vi "horizontal mag adjust.vi"(8 "y":bool=TRUE, 9 "x":bool=TRUE, 10 "2D mag correct":dbl, 11 "Array in":u16[][](array[numeric])) -> (3 "Array out":u16[][](array[numeric]))   [LabVIEW 2024]
uses:
  <vilib>/vision/NI_Vision_Development_Module.lvlib
panel:
  in  "Interpolation Type":u32(ring)=1 items=["Zero Order", "Bi-Linear", "Quadratic", "Cubic Spline"]
  out "x-y":dbl
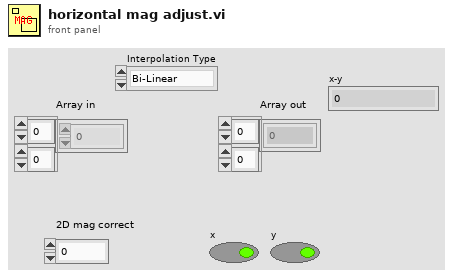
[diagram p1: front panel]
types:
  T1 = typedef "Image Type" = u32
  T2 = typedef "IMAQ Image.ctl" = refnum<image>
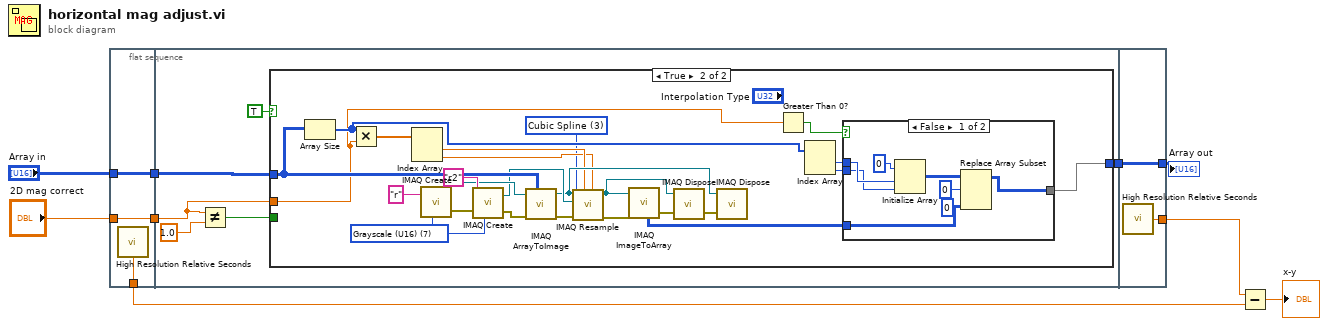
[diagram p0: block diagram]
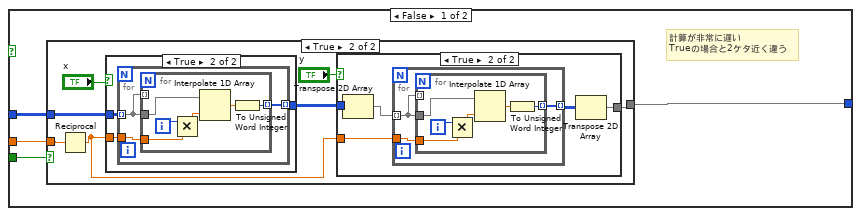
[diagram p2: hidden frame]
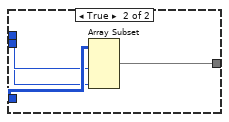
[diagram p6: hidden frame]
diagram:
  n1 = flat-sequence {
    tunnel: "2D mag correct" -> [w11]
    tunnel: "Array in" -> [w12]
    tunnel: [w12] -> w7
    tunnel: [w11] -> w6
    tunnel: [w10] -> w4
    tunnel: [w16] -> w8
    tunnel: w7 -> [w15]
    tunnel: w6 -> [w14]
    tunnel: [w97] -> w2
    tunnel: w8 -> [w97]
    tunnel: [w96] -> w5
    frame #0 {
      n2 = call <vilib>:"High Resolution Relative Seconds.vi"() -> ("relative seconds"=w10:dbl)
    }
    frame #1 {
      n3 = Not Equal?(x=w14, y=1.0) -> (x != y?=w18:bool)
      n4 = case shown="True" TRUE {
        tunnel: w18 -> [w22 _]
        tunnel: [w21 w65] -> w16
        tunnel: w15 -> [w20 w80]
        tunnel: w14 -> [w19 w60]
        frame False {
          # "計算が非常に遅い\nTrueの場合と2ケタ近く違う"
          n5 = case shown="True" w22 {
            tunnel: w20 -> [w23 w30]
            tunnel: [w23 w28] -> w21
            tunnel: w19 -> [_ w25]
            frame False {
            }
            frame True {
              n6 = Reciprocal(x=w25) -> (1/x=w24:dbl)
              n7 = case shown="True" "x" {
                tunnel: w30 -> [w31 w34]
                tunnel: [w31 w33] -> w29
                tunnel: w24 -> [_ w32]
                frame False {
                }
                frame True {
                  n8 = for {
                    tunnel: w34 -> [w36] mode=indexing
                    tunnel: w32 -> [w37]
                    tunnel: [w35] -> w33 mode=indexing
                    n9 = for {
                      tunnel: w36 -> [w41]
                      tunnel: w37 -> [w42]
                      tunnel: [w38] -> w35 mode=indexing
                      tunnel: w36 -> [_] mode=indexing
                      i -> [w43]
                      n10 = Multiply(x=w43, y=w42) -> (x*y=w40:dbl)
                      n11 = Interpolate 1D Array(1:w40, 2:w41) -> (0:w39:dbl)
                      n12 = To Unsigned Word Integer(number=w39) -> (unsigned 16bit integer=w38:u16)
                    }
                  }
                }
              }
              n13 = case shown="True" "y" {
                tunnel: w29 -> [w44 w49]
                tunnel: [w44 w46] -> w28
                tunnel: w24 -> [_ w45]
                frame False {
                }
                frame True {
                  n14 = Transpose 2D Array(2D array=w49) -> (transposed array=w48:u16[][])
                  n15 = for {
                    tunnel: w48 -> [w51] mode=indexing
                    tunnel: w45 -> [w52]
                    tunnel: [w50] -> w47 mode=indexing
                    n16 = for {
                      tunnel: w51 -> [w56]
                      tunnel: w52 -> [w57]
                      tunnel: [w53] -> w50 mode=indexing
                      tunnel: w51 -> [_] mode=indexing
                      i -> [w58]
                      n17 = Multiply(x=w58, y=w57) -> (x*y=w55:dbl)
                      n18 = Interpolate 1D Array(1:w55, 2:w56) -> (0:w54:dbl)
                      n19 = To Unsigned Word Integer(number=w54) -> (unsigned 16bit integer=w53:u16)
                    }
                  }
                  n20 = Transpose 2D Array(2D array=w47) -> (transposed array=w46:u16[][])
                }
              }
            }
          }
        }
        frame True {
          w59 = u32 3 items=["Zero Order", "Bi-Linear", "Quadratic", "Cubic Spline"] ("Interpolation Type")
          w76 = T1 7 items=["Grayscale (U8)", "Grayscale (I16)", "Grayscale (SGL)", "Complex (CSG)", "RGB (U32)", "HSL (U32)", "RGB (U64)", "Grayscale (U16)"] ("Image Type")
          n21 = Array Size(array=w80) -> (size(s)=w64:i32[])
          n22 = Multiply(x=w64, y=w60) -> (x*y=w81:dbl[])
          n23 = Index Array(array=w81) -> (element #1=w67:dbl, element #2=w66:dbl)  [unwired: 2 in]
          n24 = call "IMAQ Create"("Image Name"="r", "Image Type"=w76) -> ("New Image"=w74:T2, "error out"=w77:errorcluster)  [unwired: 3 in]
          n25 = call "IMAQ Create"("Image Name"="r2", "Image Type"=w76, "error in (no error)"=w77) -> ("New Image"=w71:T2, "error out"=w75:errorcluster)  [unwired: 2 in]
          n26 = call "IMAQ ArrayToImage"("Image Pixels (U16)"=w80, "error in (no error)"=w75, "Image"=w74) -> ("error out"=w73:errorcluster, "Image Out"=w69:T2)  [unwired: 7 in]
          n27 = call "IMAQ Resample"("X Resolution"=w66, "Y Resolution"=w67, "error in (no error)"=w73, "Interpolation Type"=w59, "Image Dst"=w71, "Image Src"=w69) -> ("error out"=w72:errorcluster, "Image Dst Out"=w70:T2)  [unwired: 4 in]
          n28 = call "IMAQ ImageToArray"("error in (no error)"=w72, "Image"=w70) -> ("Image Pixels (U16)"=w68:u16[][], "error out"=w83:errorcluster)  [unwired: 2 in, 3 out]
          n29 = call "IMAQ Dispose"("Image"=w70, "error in (no error)"=w83) -> ("error out"=w79:errorcluster)  [unwired: 4 in]
          n30 = call "IMAQ Dispose"("Image"=w69, "error in (no error)"=w79) -> ()  [unwired: 4 in, 1 out]
          n31 = Greater Than 0?(x=w60) -> (x > 0?=w61:bool)
          n32 = Index Array(array=w64) -> (element #1=w63:i32, element #2=w62:i32)  [unwired: 2 in]
          n33 = case shown="False" w61 {
            tunnel: w68 -> [w87 w95]
            tunnel: [w84 w94] -> w65
            tunnel: w63 -> [w90 w93]
            tunnel: w62 -> [w89 w92]
            frame False {
              n34 = Initialize Array(0, w90, w89) -> (w88:i32[][])
              n35 = Replace Array Subset(array=w88, new element=w87, index (row)=0, index (col)=0 ("disabled index (col)")) -> (w84:i32[][])
            }
            frame True {
              n36 = Array Subset(array=w95, length (row)=w93, length (col)=w92) -> (w94:u16[][])  [unwired: 2 in]
            }
          }
        }
      }
    }
    frame #2 {
      n37 = call <vilib>:"High Resolution Relative Seconds.vi"() -> ("relative seconds"=w96:dbl)
    }
  }
  n38 = Subtract(x=w5, y=w4) -> (x-y=→"x-y":dbl)
  "Array out" <- w2
